vi "Configure Active Meter.vi"(0 "VISA resource name":refnum<visa-resource-name>, 5 "Active Meter (0:Frequency)":u16(ring) items=["Frequency", "Current", "Power", "Active Reactive Current", "Creast Factor", "Peak Current", "Active Apparent Power", "Power Factor", "Cycle"], 11 "error in (no error)":errorcluster) -> (4 "VISA resource name out":refnum<visa-resource-name>, 15 "error out":errorcluster)   [LabVIEW 2016, in "APT 300XAC Series.lvlib"]
doc: "Sets <B>active meter</B> on the display of the power source instrument.\n\nAC Range Program mode:\nValue = 0-8; 0=F, 1=A, 2=P, 3=Q, 4=CF, 5=AP, 6=VA, 7=PF, 8=CYCLE\n\nAC Range Manual mode\nValue = 0-7; 0=F, 1=A, 2=P, 3=Q, 4=CF, 5=AP, 6=VA, 7=PF\n\nDC Range Program mode\nValue = 1,2,8; 1=A, 2=P, 8=CYCLE\n\nDC Range Manual mode\nValue = 1,2,8; 1=A, 2=P"
uses:
  APT 300XAC Series.lvlib
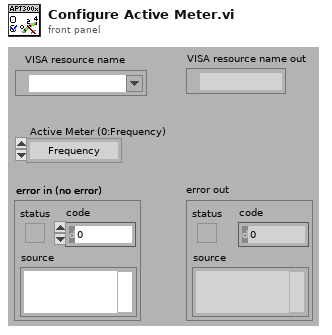
[diagram p1: front panel]
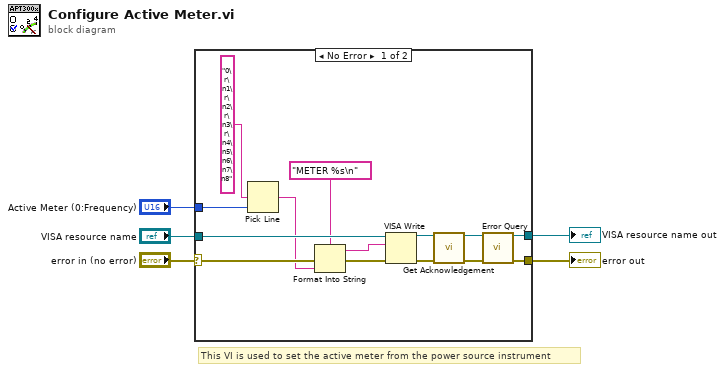
[diagram p0: block diagram]
diagram:
  # "This VI is used to set the active meter from the power source instrument"
  n1 = case shown="No Error" "error in (no error)" {
    selector: "error in (no error)" -> [w12 w20]
    tunnel: "VISA resource name" -> [w19 w21]
    tunnel: "Active Meter (0:Frequency)" -> [w17 _]
    tunnel: [w16 w21] -> w3
    tunnel: [w15 w20] -> w2
    frame No Error {
      n2 = Pick Line(multi-line string="0\r\n1\r\n2\r\n3\r\n4\n5\n6\n7\n8" ("options"), line index=w17) -> (output string=w10:string)  [unwired: 1 in]
      n3 = Format Into String(format string="METER %s\n" ("command"), error in=w12, w10) -> (resulting string=w13:string, error out=w11:errorcluster)  [unwired: 1 in]
      n4 = VISA Write(VISA resource name=w19, write buffer=w13, error in (no error)=w11) -> (VISA resource name out=w8:refnum<visa-resource-name>, error out=w7:errorcluster)  [unwired: 1 out]
      n5 = call "Get Acknowledgement.vi"("VISA resource name"=w8, "error in (no error)"=w7) -> ("VISA resource name out"=w9:refnum<visa-resource-name>, "error out"=w6:errorcluster)  [unwired: 12 in]
      n6 = call "Error Query.vi"("VISA resource name"=w9, "error in (no error)"=w6) -> ("VISA resource name out"=w16:refnum<visa-resource-name>, "error out"=w15:errorcluster)  [unwired: 10 in, 2 out]
    }
    frame Error {
    }
  }
  "VISA resource name out" <- w3
  "error out" <- w2
